vi "灯值状态读取.vi"(8 "error in (no error)":errorcluster) -> (0 "error out":errorcluster, 3 "状态值":cluster{"校准状态":u16, "当前阻值":u16, "当前光强":u16} {"校准状态" items=["空闲", "校准中"]})   [LabVIEW 2016, in "斯坦道CODcr.lvlib"]
uses:
  <vilib>/Plasmionique/MB Master/MB Master.lvlib
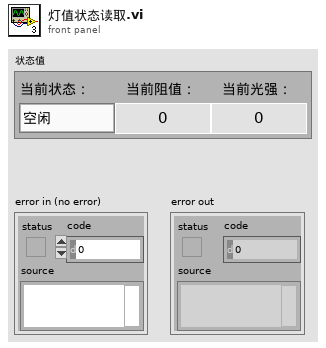
[diagram p1: front panel]
types:
  T1 = cluster{"WORD[0]":u16, "WORD[1]":u16, "WORD[2]":u16}
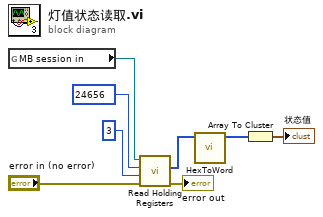
[diagram p0: block diagram]
diagram:
  n1 = global read "VAR总磷总氮全局变量.vi" "MB session in"() -> (w8:refnum<class "MB_Master.lvclass">)
  n2 = call <vilib>:"Read Holding Registers.vi"("error in (no error)"="error in (no error)", "quantity"=u16 3, "starting address"=u16 24656, "MB session in"=w8) -> ("error out"=→"error out":errorcluster, "Registers"=w3:u16[])  [unwired: 5 in, 1 out]
  n3 = call "HexToWord.vi"("数组"=w3) -> ("WORD"=w2:u16[])  [unwired: 10 in]
  n4 = Array To Cluster(array=w2) -> (cluster=→"状态值":T1)
